vi "Configure Upper Pressure Limit.vi"(5 "Retry Attempts (0)":i32 min=0, 8 "error in":errorcluster, 10 "Upper Pressure Limit":i32, 11 "VISA resource name":refnum<visa-resource-name>) -> (0 "error out":errorcluster, 3 "VISA resource name out":refnum<visa-resource-name>)   [LabVIEW 2020, in "ChromTech Series III Pump.lvlib"]
doc: "Configures the flow rate using up to 5 digits. If the entered value exceeds the maximum allowable flow rate of the pump, the flow rate will be automatically set to the maximum allowable flow rate. The maximum allowable flow rate can be found using the Get Maximum Flow Rate VI and the current flow rate can be found using the Get Current Flow Rate VI or Get Current Conditions VI"
uses:
  <instrlib>/ChromTech Series III Pump/ChromTech Series III Pump.lvlib
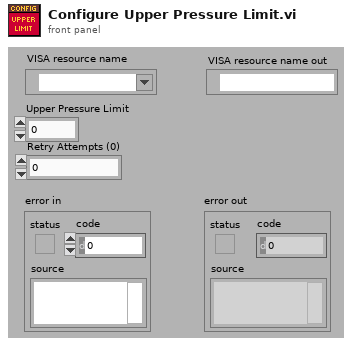
[diagram p1: front panel]
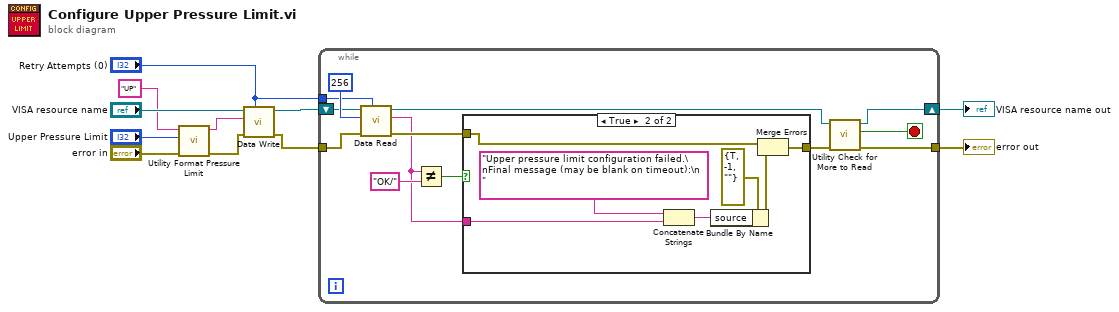
[diagram p0: block diagram]
diagram:
  n1 = call <instrlib>:"Utility Format Pressure Limit.vi"("error in (no error)"="error in", "Pressure Limit"="Upper Pressure Limit", "Pressure Limit Command"="UP") -> ("error out"=w7:errorcluster, "Formatted Command"=w6:string)  [unwired: 7 in]
  n2 = call <instrlib>:"Data Write.vi"("Retry Attempts (0)"="Retry Attempts (0)", "error in (no error)"=w7, "Command"=w6, "VISA Refnum in"="VISA resource name") -> ("error out"=w10:errorcluster, "VISA Refnum out"=w5:refnum<visa-resource-name>)  [unwired: 6 in]
  n3 = while {
    shift-right: [w14] -> w9
    shift-left: w5 -> [w22]
    tunnel: "Retry Attempts (0)" -> [w13]
    tunnel: w10 -> [w24]
    tunnel: [w16] -> w2
    stop <- w12 stop-if-true
    n4 = call <instrlib>:"Data Read.vi"("Retry Attempts (0)"=w13, "error in (no error)"=w24, "Bytes to read"=256, "VISA Refnum in"=w22) -> ("error out"=w21:errorcluster, "read buffer"=w17:string, "VISA Refnum out"=w15:refnum<visa-resource-name>)  [unwired: 5 in]
    n5 = Not Equal?(x=w17, y="OK/") -> (x != y?=w19:bool)
    n6 = case shown="True" w19 {
      tunnel: [w25 w31] -> w20
      tunnel: w21 -> [w25 w30]
      tunnel: w17 -> [_ w26]
      frame False {
      }
      frame True {
        n7 = Concatenate Strings("Upper pressure limit configuration failed.\nFinal message (may be blank on timeout):\n ", w26) -> (w28:string)
        n8 = Bundle By Name(cluster=errorcluster {"status"=TRUE, "code"=-1, "source"=""} ("error out"), "source"=w28) -> (w29:errorcluster)
        n9 = Merge Errors(w30, w29) -> (w31:errorcluster)
      }
    }
    n10 = call <instrlib>:"Utility Check for More to Read.vi"("error in (no error)"=w20, "VISA Refnum in"=w15) -> ("error out (unchanged)"=w16:errorcluster, "More to read?"=w12:bool, "VISA Refnum out"=w14:refnum<visa-resource-name>)  [unwired: 7 in]
  }
  "VISA resource name out" <- w9
  "error out" <- w2
